vi "GA_Set_Parameters.vi"(7 "Dimension":i32, 8 "error in (no error)":errorcluster, 9 "Number of Generations":i32, 10 "Front Panel Menu":T1={"Crossover Probability"=0.75, "Mutation Probability"=0.2, "Population Size"=80, "Strategy"=enum."Normal", "Plot Type"=enum."No Plot"}, 11 "GA in":refnum<class "GA.lvclass">) -> (0 "error out":errorcluster, 3 "GA out":refnum<class "GA.lvclass">)   [LabVIEW 2013, in "GA.lvclass"]
uses:
  GA.lvclass
  Controls/Front Panle Menu.ctl
  Controls/Strategy.ctl
  Controls/Plot Type.ctl
  Controls/Solution.ctl
  Controls/Population Statistics.ctl
  GA.lvclass/GA.ctl
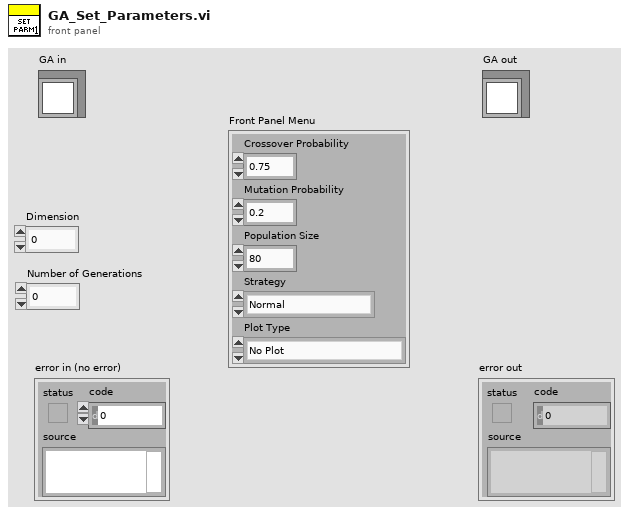
[diagram p1: front panel]
types:
  T1 = typedef "Front Panle Menu.ctl" = cluster{"Crossover Probability":dbl, "Mutation Probability":dbl, "Population Size":u8, "Strategy":T2, "Plot Type":T3}
  T2 = typedef "Strategy.ctl" = enum16{"Normal", "Ellitist 1", "Elitist 2"}
  T3 = typedef "Plot Type.ctl" = enum16{"No Plot", "Min Max Mean Plot", "Gannt Chart"}
  T4 = typedef "Population Statistics.ctl" = cluster{"Min":u16, "Max":u16, "Mean":dbl}
  T5 = typedef "Solution.ctl" = cluster{"Schedule":u16[], "Fitness":u16, "Fitness Valid?":bool}
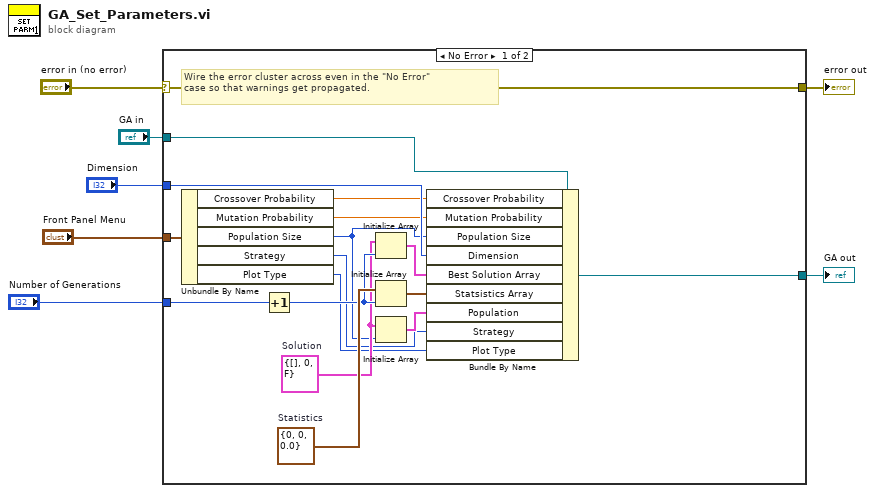
[diagram p0: block diagram]
diagram:
  n1 = case shown="No Error" "error in (no error)" {
    selector: "error in (no error)" -> [w24 w26]
    tunnel: [w24 w26] -> w6
    tunnel: [w22 w25] -> w4
    tunnel: "GA in" -> [w23 w25]
    tunnel: "Dimension" -> [w21 _]
    tunnel: "Number of Generations" -> [w17 _]
    tunnel: "Front Panel Menu" -> [w13 _]
    frame No Error {
      w19 = T4 {"Min"=0, "Max"=0, "Mean"=0.0}  # Statistics
      w15 = T5 {"Schedule"=[], "Fitness"=0, "Fitness Valid?"=FALSE}  # Solution
      # "Wire the error cluster across even in the \"No Error\"\ncase so that warnings get propagated."
      n2 = Unbundle By Name(w13) -> ("Crossover Probability"=w12:dbl, "Mutation Probability"=w11:dbl, "Population Size"=w10:u8, "Strategy"=w9:T2, "Plot Type"=w8:T3)
      n3 = Increment(x=w17) -> (x+1=w16:i32)
      n4 = Initialize Array(w15, w16) -> (w20:T5[])
      n5 = Initialize Array(w19, w16) -> (w18:T4[])
      n6 = Initialize Array(w15, w10) -> (w14:T5[])
      n7 = Bundle By Name(cluster=w23, "Crossover Probability"=w12, "Mutation Probability"=w11, "Population Size"=w10, "Dimension"=w21, "Best Solution Array"=w20, "Statsistics Array"=w18, "Population"=w14, "Strategy"=w9, "Plot Type"=w8) -> (w22:refnum<class "GA.lvclass">)
    }
    frame Error {
    }
  }
  "error out" <- w6
  "GA out" <- w4
